vi "Read Class Data.vi"(0 "System Exec Data in":refnum<class "System Exec Data.lvclass">, 11 "error in (no error)":errorcluster) -> (3 "alias":string, 4 "System Exec Data out":refnum<class "System Exec Data.lvclass">, 6 "standard output":string, 8 "standard error":string, 10 "return code":i32, 15 "error out":errorcluster)   [LabVIEW 2020, in "ProjectBuilder.lvlib" / "System Exec Data.lvclass"]
doc: "Read the status string from the private data."
uses:
  System Exec Data.lvclass
  System Exec Data.lvclass/System Exec Data.ctl
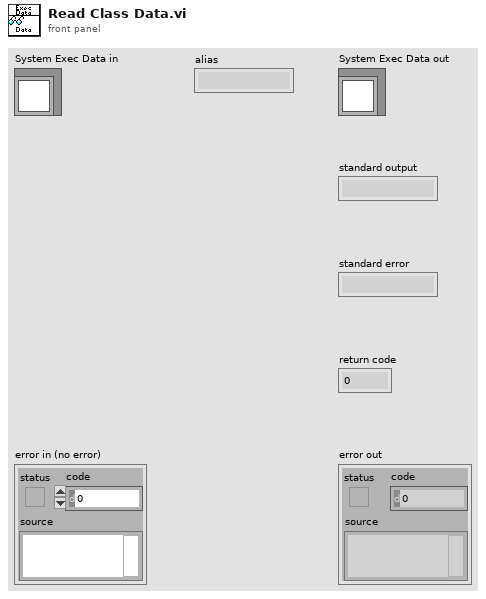
[diagram p1: front panel]
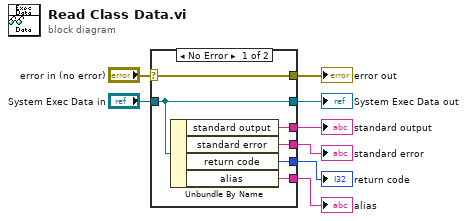
[diagram p0: block diagram]
diagram:
  n1 = case shown="No Error" "error in (no error)" {
    selector: "error in (no error)" -> [w14 w15]
    tunnel: [w14 w15] -> w7
    tunnel: [w13 w16] -> w5
    tunnel: "System Exec Data in" -> [w13 w16]
    tunnel: [w12 _] -> w4
    tunnel: [w11 _] -> w3
    tunnel: [w10 _] -> w2
    tunnel: [w9 _] -> w1
    frame No Error {
      n2 = Unbundle By Name(w13) -> ("standard output"=w10:string, "standard error"=w11:string, "return code"=w12:i32, "alias"=w9:string)
    }
    frame Error {
    }
  }
  "error out" <- w7
  "System Exec Data out" <- w5
  "standard output" <- w2
  "standard error" <- w3
  "return code" <- w4
  "alias" <- w1
